vi "DAQ.vi"() -> ()   [LabVIEW 2018]
uses:
  <vilib>/DAQmx/write.llb/DAQmx Write (Digital Bool 1Line 1Point).vi
  <vilib>/DAQmx/read.llb/DAQmx Read (Analog Wfm 1Chan NSamp).vi
  <vilib>/DAQmx/miscellaneous.llb/DAQmx Fill In Error Info.vi
panel:
  out "TimeStep":dbl
  out "Time":dbl
  out "Mahtuvus ( F )":dbl
  out "Takistus (Oom)":dbl
  out "RC":dbl
  in  "stop":bool
  out "Charge/Discharge":waveform(dbl)[](graph)
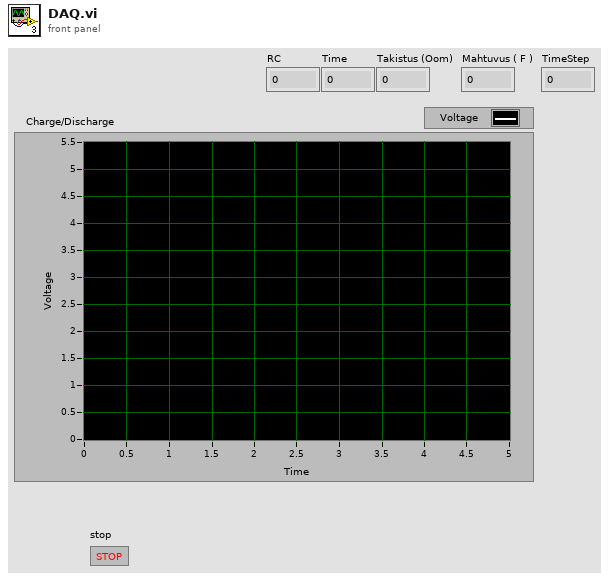
[diagram p1: front panel]
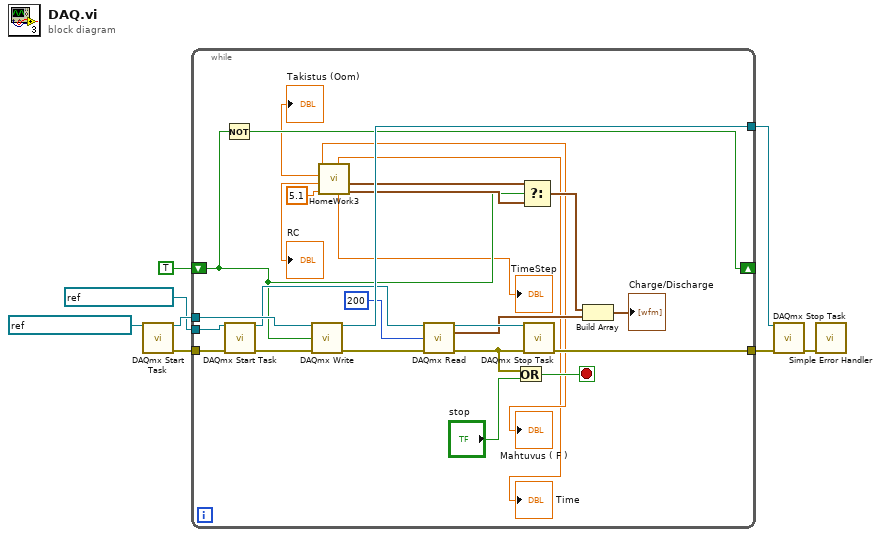
[diagram p0: block diagram]
diagram:
  n1 = call <vilib>:"DAQmx Start Task.vi"("task/channels in"=refnum<k21> "MyDigitalOutTask") -> ("task out"=w7:refnum<k21>, "error out"=w3:errorcluster)  [unwired: 13 in]
  n2 = while {
    tunnel: w7 -> [w34]
    tunnel: [w32] -> w6
    shift-right: [w28] -> _
    shift-left: TRUE -> [w11]
    tunnel: refnum<k21> "MyVoltageTask" ("task/channels in") -> [w26]
    tunnel: w3 -> [w24]
    tunnel: [w21] -> w2
    stop <- w29 stop-if-true
    n3 = Not(x=w11) -> (.not. x?=w28:bool)
    n4 = call <vilib>:"DAQmx Start Task.vi"("task/channels in"=w26, "error in"=w24) -> ("task out"=w25:refnum<k21>, "error out"=w23:errorcluster)  [unwired: 12 in]
    n5 = call-poly <vilib>:"DAQmx Write.vi"("task/channels in"=w34, "data"=w11, "error in"=w23) -> ("task out"=w32:refnum<k21>, "error out"=w33:errorcluster)  [unwired: 10 in, 1 out]
    n6 = call "HomeWork3.vi"("Voltage"=5.1) -> ("Mahtuvus ( F )"=→"Mahtuvus ( F )":dbl, "Takistus (Oom)"=→"Takistus (Oom)":dbl, "RC"=→"RC":dbl, "Time"=→"Time":dbl, "TimeStep"=→"TimeStep":dbl, "Discharging waveform"=w18:waveform(dbl), "Charging waveform"=w19:waveform(dbl))  [unwired: 1 in, 2 out]
    n7 = call-poly <vilib>:"DAQmx Read.vi"("task/channels in"=w25, "number of samples per channel"=200, "error in"=w33) -> ("task out"=w22:refnum<k21>, "data"=w15:waveform(dbl), "error out"=w30:errorcluster)  [unwired: 10 in]
    n8 = Or(x=w30, y="stop") -> (x .or. y?=w29:bool)
    n9 = Select(t=w18, s=w11, f=w19) -> (s? t:f=w17:waveform(dbl))
    n10 = call <vilib>:"DAQmx Stop Task.vi"("task/channels in"=w22, "error in"=w30) -> ("error out"=w21:errorcluster)  [unwired: 12 in, 1 out]
    n11 = Build Array(w17, w15) -> (→"Charge/Discharge":waveform(dbl)[])
  }
  n12 = call <vilib>:"DAQmx Stop Task.vi"("task/channels in"=w6, "error in"=w2) -> ("error out"=w5:errorcluster)  [unwired: 12 in, 1 out]
  n13 = call <vilib>:"Simple Error Handler.vi"("error in (no error)"=w5) -> ()  [unwired: 4 in, 5 out]
